vi "CliFullUpload.vi"(0 "ref in":u64, 5 "BlockType":i32(ring)=56 items=["OB"=56, "DB"=65, "SDB"=66, "FC"=67, "SFC"=68, "FB"=69, "SFB"=70], 7 "Block Number":i32=1, 9 "data in":string, 11 "error in (no error)":errorcluster) -> (4 "ref out":u64, 6 "Result":i32, 8 "SizeGet":i32, 10 "data out":string, 15 "error out":errorcluster)   [LabVIEW 2020, in "Snap7.lvlib"]
uses:
  Snap7.lvlib
  windows/lv_snap7.dll
panel:
  in  "var SizeGet":i32
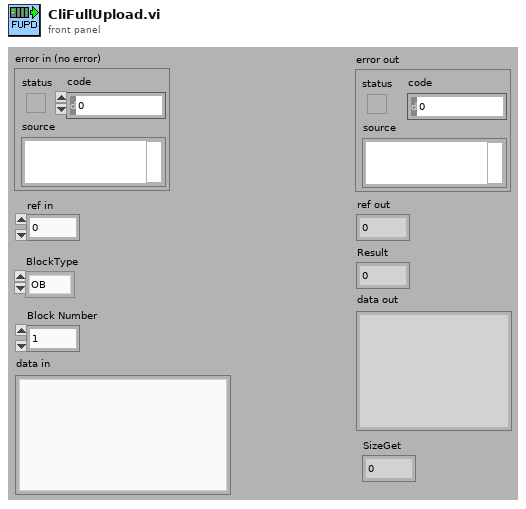
[diagram p1: front panel]
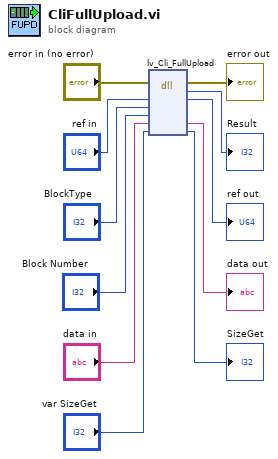
[diagram p0: block diagram]
diagram:
  n1 = dll-call lib="PTH2iabs CUsersFeng项目HLCEPS300-1老性能试验台SourcesSnap7libwindowslv_snap7.dll" fn="lv_Cli_FullUpload"(error in="error in (no error)", "Client"="ref in", "BlockType"="BlockType", "BlockNumber"="Block Number", "pUsrData"="data in", "SizeGet"="var SizeGet") -> (error out=→"error out":errorcluster, "return type"=→"Result":i32, "Client"=→"ref out":u64, "pUsrData"=→"data out":string, "SizeGet"=→"SizeGet":i32)  [unwired: 4 in, 1 out]
